vi "VI Tree - variantconfig__ogtk.vi"() -> ()   [LabVIEW 2017]
uses:
  <vilib>/Utility/config.llb/Config Data RefNum.ctl
  <vilib>/Utility/config.llb/NI_LVConfig.lvlib
panel:
  in  "VI ref":refnum<vi>
  in  "refnum":T1
types:
  T1 = typedef "NI_LVConfig.lvlib/Config Data RefNum.ctl" = refnum<k1>
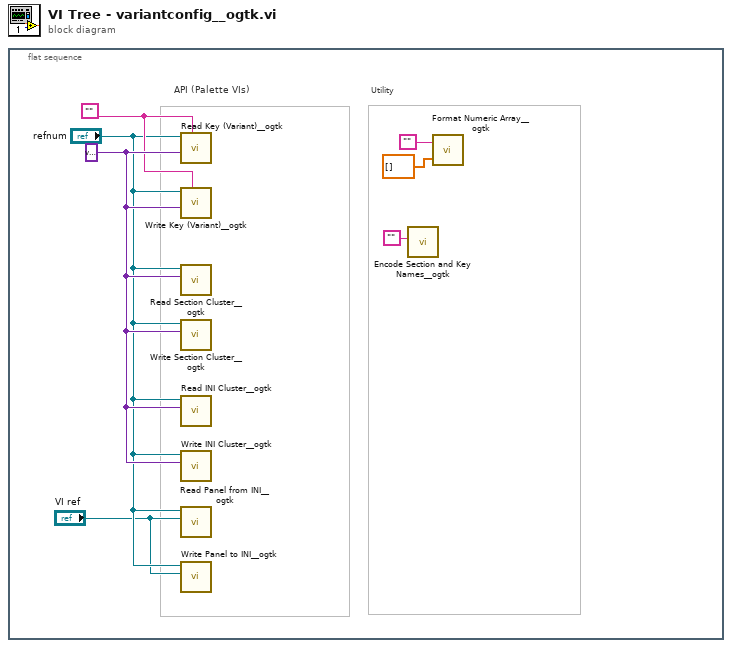
[diagram p0: block diagram]
diagram:
  n1 = flat-sequence {
    frame #0 {
      w7 = variant ("type")
      w6 = ""
      # "Utility"
      # "API (Palette VIs)"
      n2 = call <userlib>:"Read Key (Variant)__ogtk.vi"("section"=w6, "type"=w7, "refnum"="refnum") -> ()  [unwired: 5 in, 4 out]
      n3 = call <userlib>:"Write Key (Variant)__ogtk.vi"("section"=w6, "key-value"=w7, "refnum"="refnum") -> ()  [unwired: 7 in, 2 out]
      n4 = call <userlib>:"Read Section Cluster__ogtk.vi"("Section Formatted Cluster Type"=w7, "refnum"="refnum") -> ()  [unwired: 5 in, 5 out]
      n5 = call <userlib>:"Write Section Cluster__ogtk.vi"("Section Formatted Cluster"=w7, "refnum"="refnum") -> ()  [unwired: 8 in, 2 out]
      n6 = call <userlib>:"Read INI Cluster__ogtk.vi"("INI Fomatted Cluster Type"=w7, "refnum"="refnum") -> ()  [unwired: 5 in, 5 out]
      n7 = call <userlib>:"Write INI Cluster__ogtk.vi"("INI Fomatted Cluster"=w7, "refnum"="refnum") -> ()  [unwired: 8 in, 2 out]
      n8 = call <userlib>:"Read Panel from INI__ogtk.vi"("VI ref"="VI ref", "refnum"="refnum") -> ()  [unwired: 8 in, 2 out]
      n9 = call <userlib>:"Write Panel to INI__ogtk.vi"("VI ref"="VI ref", "refnum"="refnum") -> ()  [unwired: 8 in, 2 out]
      n10 = call <userlib>:"Encode Section and Key Names__ogtk.vi"("string"="" ("format string")) -> ()  [unwired: 10 in, 1 out]
      n11 = call <userlib>:"Format Numeric Array__ogtk.vi"("Array"=dbl[] [], "format string"="") -> ()  [unwired: 1 out]
    }
  }
